vi "1_Waveform_Signal_Regression_Multi_Output(Training).vi"() -> ()   [LabVIEW 2020]
uses:
  <vilib>/Ngene/DeepLTK/Toolkit/NN_Train/Controls/NN_LR_Policy_Cfg.ctl
  <vilib>/Ngene/DeepLTK/Toolkit/NN_Train/Controls/NN_LR_Policy_Type.ctl
  <vilib>/Ngene/DeepLTK/Toolkit/NN_Train/Controls/NN_Train_Session_Data.ctl
  <vilib>/Ngene/DeepLTK/Toolkit/NN_Train/Controls/NN_Train_Params.ctl
  <vilib>/Ngene/DeepLTK/Toolkit/NN_Train/Controls/NN_Train_Optimizer.ctl
  <vilib>/Ngene/DeepLTK/Toolkit/NN_Train/Controls/NN_Train_Data_Sampling.ctl
  <vilib>/Ngene/DeepLTK/Toolkit/NN_Network/Controls/NN_Device.ctl
  <vilib>/Ngene/DeepLTK/Toolkit/NN_Layers/Layers/Input/Controls/NN_Layer_Config(Input1D).ctl
  <vilib>/Ngene/DeepLTK/Toolkit/NN_Layers/Layers/FC/Controls/NN_Layer_Config(FC).ctl
  <vilib>/Ngene/DeepLTK/Toolkit/NN_Activations/Controls/NN_Activation_Type.ctl
  <vilib>/Ngene/DeepLTK/Toolkit/NN_Layers/Controls/NN_Layer_Init_Params.ctl
  <vilib>/Ngene/DeepLTK/Toolkit/NN_Layers/Controls/NN_Layer_Weight_Init_Type.ctl
  <vilib>/Ngene/DeepLTK/Toolkit/NN_Network/Controls/NN_Save_Before_Destroy_Options.ctl
  <vilib>/Ngene/DeepLTK/Toolkit/NN_Layers/Layers/Input/NN_Layer_Create(Input1D).vi
  <vilib>/Ngene/DeepLTK/Toolkit/NN_Layers/Layers/FC/NN_Layer_Create(FC).vi
  <vilib>/Ngene/DeepLTK/Toolkit/NN_Train/Loss_Functions/NN_Set_Loss(MSE).vi
  <vilib>/Ngene/DeepLTK/Toolkit/NN_Network/subVIs/NN_Predict/NN_Predict(In1D_Out1D).vi
  <vilib>/Ngene/DeepLTK/Toolkit/NN_Train/Eval_Loss/NN_Eval_Test_Error_Loss/NN_Eval(In1D_Out1D).vi
  <vilib>/Ngene/DeepLTK/Toolkit/Deep_Learning_Toolkit_by_Ngene.lvlib
  <vilib>/ptbypt/NI_PtbyPt.lvlib
panel:
  out "Training Loss":sgl=0.0060925223 format="%#.6g"
  in  "Eval":bool
  out "Loss Graphs":cluster{"mean":dbl, "mean":dbl}(graph)={"mean"=0.014923217580653727, "mean"=0.03191827982664108}
  in  "NN_Device":T1=enum."GPU"
  out "Test Loss":sgl=0.03191828 format="%#.6g"
  in  "Stop Training":bool
  in  "NN_Train_Params":T2={"Optimizer"=enum."Adam", "Beta_1"=0.9, "Beta_2"=0.999, "Weight Decay(L1)"=1e-08, "Weight Decay(L2)"=1e-08, "Data_Sampling"=enum."Random"}
  out "Session Data":T5={"Epochs"=39.18592, "Tot_Iter"=30614, "LR"=6.25e-05, "LR_iter"=30615} {"LR" format="%#_3g"}
  in  "LR Update Policy":T6={"Policy_Type"=enum."Step", "LR0"=0.001, "k"=5.0, "WarmUp_Policy"=enum."Ramp", "WarmUp_Iter"=1000, "WarmUp_Ratio"=100.0} {"WarmUp_Ratio" min=1; "WarmUp_Iter" min=1; "LR0" format="%.7f"}
  # "Overview: This example demonstrates the usage of Deep Learning Toolkit for solving multiple output waveform signal regression problem. Specifically, a model is trained to predict multiple characteristic properties of a waveform, such as frequency, amplitude, phase, and DC offset..\nRequirements: DeepLTK - Deep Learning Toolkit for LabVIEW.\nInstructions:\n1.  Run the VI with current configuration of the training parameters and Learning Rate update policy.\n2. Observe how the training loss is decreasing.\n3. Press the \"Stop Training\" when the loss is not decreasing any more.\nMore Examples:  https://github.com/ngenehub/deepltk_examples"
  # "Waveform Signal Regression (Frequency Prediction) - Training"
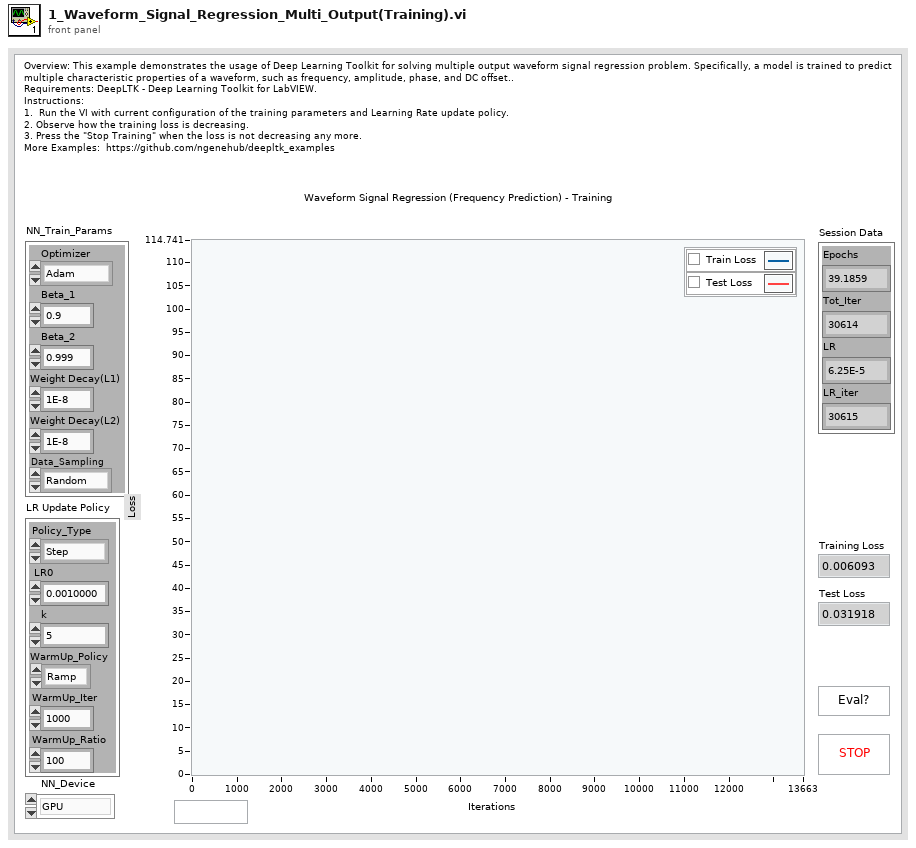
[diagram p1: front panel]
types:
  T1 = typedef "Deep_Learning_Toolkit_by_Ngene.lvlib/NN_Device.ctl" = enum16{"CPU", "GPU"}
  T2 = typedef "Deep_Learning_Toolkit_by_Ngene.lvlib/NN_Train_Params.ctl" = cluster{"Optimizer":T3, "Beta_1":sgl, "Beta_2":sgl, "Weight Decay(L1)":sgl, "Weight Decay(L2)":sgl, "Data_Sampling":T4}
  T3 = typedef "Deep_Learning_Toolkit_by_Ngene.lvlib/NN_Train_Optimizer.ctl" = enum16{"SGD", "Adam", "Adagrad", "Adadelta", "RMSProp", "Nesterov"}
  T4 = typedef "Deep_Learning_Toolkit_by_Ngene.lvlib/NN_Train_Data_Sampling.ctl" = enum16{"Random", "Sequential"}
  T5 = typedef "Deep_Learning_Toolkit_by_Ngene.lvlib/NN_Train_Session_Data.ctl" = cluster{"Epochs":sgl, "Tot_Iter":i32, "LR":sgl, "LR_iter":i32}
  T6 = typedef "Deep_Learning_Toolkit_by_Ngene.lvlib/NN_LR_Policy_Cfg.ctl" = cluster{"Policy_Type":T7, "LR0":dbl, "k":sgl, "WarmUp_Policy":enum16{"Step", "Ramp"}, "WarmUp_Iter":i32, "WarmUp_Ratio":sgl}
  T7 = typedef "Deep_Learning_Toolkit_by_Ngene.lvlib/NN_LR_Policy_Type.ctl" = enum16{"Manual", "Step", "Exp", "1/t"}
  T8 = typedef "Deep_Learning_Toolkit_by_Ngene.lvlib/NN_Layer_Config(FC).ctl" = cluster{"Name":string, "Size":i32, "BN":bool, "Activation":T9, "Init_Params":T10, "Custom_Params":string}
  T9 = typedef "Deep_Learning_Toolkit_by_Ngene.lvlib/NN_Activation_Type.ctl" = enum16{"Sigmoid", "ReLU", "LReLU", "ReLU6", "tanh", "Swish", "Mish", "None"}
  T10 = typedef "Deep_Learning_Toolkit_by_Ngene.lvlib/NN_Layer_Init_Params.ctl" = cluster{"Init_Type":T11, "Value":sgl}
  T11 = typedef "Deep_Learning_Toolkit_by_Ngene.lvlib/NN_Layer_Weight_Init_Type.ctl" = enum16{"Const", "Uniform", "Gaussian", "Xavier"}
  T12 = typedef "Deep_Learning_Toolkit_by_Ngene.lvlib/NN_Save_Before_Destroy_Options.ctl" = cluster{"CFG?":bool, "Weights?":bool, "Render?":bool}
  T13 = typedef "Deep_Learning_Toolkit_by_Ngene.lvlib/NN_Layer_Config(Input1D).ctl" = cluster{"Name":string, "Size":i32}
  T14 = typedef "Deep_Learning_Toolkit_by_Ngene.lvlib/NN_DataSets_All(In1D_Out1D).ctl" = cluster{"Train":T15, "Validation":T15, "Test":T15}
  T15 = typedef "Deep_Learning_Toolkit_by_Ngene.lvlib/NN_DataSet(In1D_Out1D).ctl" = cluster{"Inputs Ref.":T16, "Outputs Ref.":T16, "Dims_In":i32, "Dataset_Size":i32, "Outputs_idx Ref.":T17, "Dims_Out":i32, "Labels":string[], "File Paths":path[]}
  T16 = typedef "Deep_Learning_Toolkit_by_Ngene.lvlib/NN_Data_ref(2D_SGL).ctl" = refnum<data-value>
  T17 = typedef "Deep_Learning_Toolkit_by_Ngene.lvlib/NN_Data_ref(1D_I32).ctl" = refnum<data-value>
  T18 = typedef "Deep_Learning_Toolkit_by_Ngene.lvlib/NN.ctl" = cluster{"Name":string, "No of Layers":i32, "mBatch":i32, "Layers":T19[], "Dimty":T20, "Dims_In":T21, "Dims_Out":T21, "Working_Dir":path, "Train?":bool, "Train_Params":T2, "LR_Update_Policy":T6, "Session Data":T5, "Ground_truth":T22, "NNg_hdls":T23, "NN_Device":T1, "GPU Id":i32, "Labels":string[], "Receptive Field":T24[], "Loss_Type":T25, "Loss_Cfg_Prms":variant}
  T19 = typedef "Deep_Learning_Toolkit_by_Ngene.lvlib/NN_Layer_ref.ctl" = refnum<data-value>
  T20 = typedef "Deep_Learning_Toolkit_by_Ngene.lvlib/NN_In_Out_Dim-ty.ctl" = enum8{"In1D_Out1D", "In3D_Out1D", "In3D_Out3D", "In3D_OutBBox"}
  T21 = typedef "Deep_Learning_Toolkit_by_Ngene.lvlib/NN_Dims(C,H,W).ctl" = cluster{"C":i32, "H":i32, "W":i32}
  T22 = typedef "Deep_Learning_Toolkit_by_Ngene.lvlib/NN_Ground_truth.ctl" = cluster{"Y":variant, "Y_idx":T17}
  T23 = typedef "Deep_Learning_Toolkit_by_Ngene.lvlib/nng_cuda_handles.ctl" = cluster{"cudnn":u64, "cublas":u64, "stream":u64, "curand":u64}
  T24 = typedef "Deep_Learning_Toolkit_by_Ngene.lvlib/NN_Dims(V,H).ctl" = cluster{"V":i32, "H":i32}
  T25 = typedef "Deep_Learning_Toolkit_by_Ngene.lvlib/NN_Loss_Type.ctl" = enum16{"None", "MSE", "CrossEntropy", "YOLO_v2"}
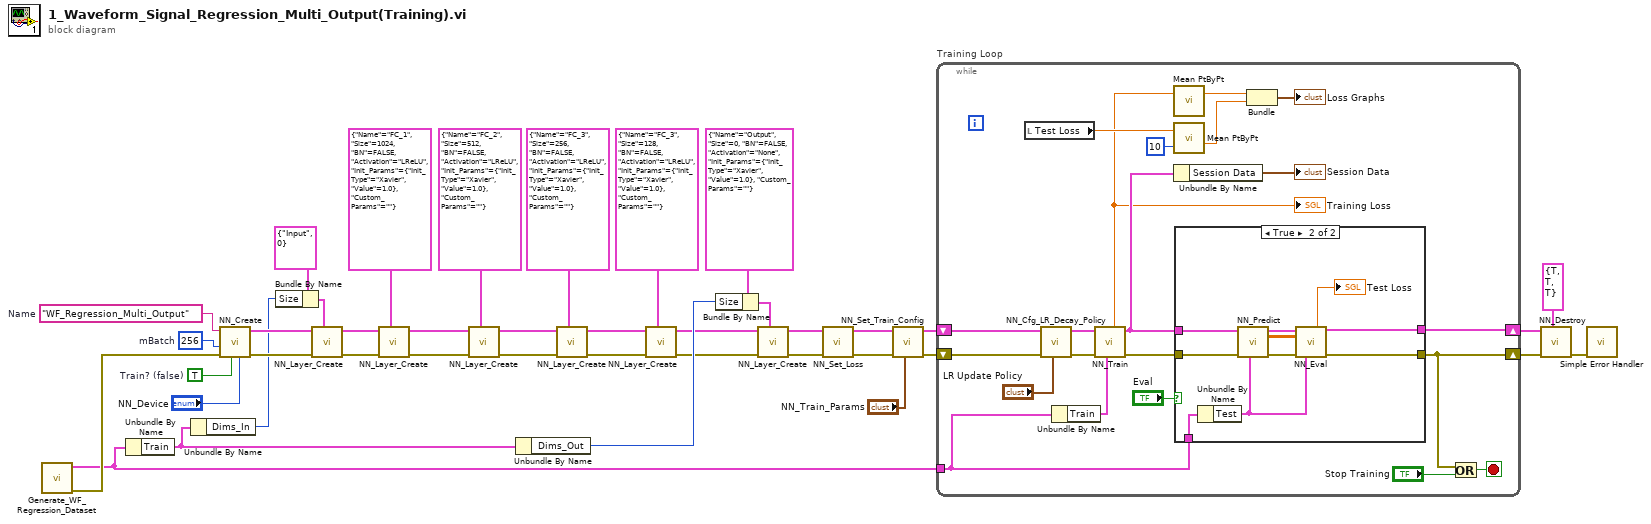
[diagram p0: block diagram]
diagram:
  w21 = "WF_Regression_Multi_Output"  # Name
  w22 = 256  # mBatch
  w23 = TRUE  # Train? (false)
  n1 = call "Generate_WF_Regression_Dataset.vi"() -> ("error out"=w32:errorcluster, "DataSets_All(In1D_Out1D)"=w8:T14)  [unwired: 10 in]
  n2 = Unbundle By Name(w8) -> ("Train"=w6:T15)
  n3 = Unbundle By Name(w6) -> ("Dims_In"=w30:i32)
  n4 = call <vilib>:"NN_Create.vi"("NN_Device"="NN_Device", "Train? (false)"=w23, "error in (no error)"=w32, "mBatch (1)"=w22, "Name"=w21) -> ("error out"=w39:errorcluster, "NN out"=w40:T18)  [unwired: 5 in]
  n5 = Bundle By Name(cluster=T13 {"Name"="Input", "Size"=0} ("Input1D_Cfg"), "Size"=w30) -> (w31:T13)
  n6 = call-poly <vilib>:"NN_Layer_Create.vi"("Input1D_Cfg"=w31, "error in (no error)"=w39, "NN in"=w40) -> ("error out"=w26:errorcluster, "NN out"=w27:T18)  [unwired: 6 in, 1 out]
  n7 = call-poly <vilib>:"NN_Layer_Create.vi"("FC_Cfg"=T8 {"Name"="FC_1", "Size"=1024, "BN"=FALSE, "Activation"=enum."LReLU", "Init_Params"={"Init_Type"=enum."Xavier", "Value"=1.0}, "Custom_Params"=""} ("FC_Cfg_1"), "error in (no error)"=w26, "NN in"=w27) -> ("error out"=w15:errorcluster, "NN out"=w16:T18)  [unwired: 6 in, 1 out]
  n8 = call-poly <vilib>:"NN_Layer_Create.vi"("FC_Cfg"=T8 {"Name"="FC_2", "Size"=512, "BN"=FALSE, "Activation"=enum."LReLU", "Init_Params"={"Init_Type"=enum."Xavier", "Value"=1.0}, "Custom_Params"=""} ("FC_Cfg_1"), "error in (no error)"=w15, "NN in"=w16) -> ("error out"=w11:errorcluster, "NN out"=w12:T18)  [unwired: 6 in, 1 out]
  n9 = Unbundle By Name(w6) -> ("Dims_Out"=w28:i32)
  n10 = call-poly <vilib>:"NN_Layer_Create.vi"("FC_Cfg"=T8 {"Name"="FC_3", "Size"=256, "BN"=FALSE, "Activation"=enum."LReLU", "Init_Params"={"Init_Type"=enum."Xavier", "Value"=1.0}, "Custom_Params"=""} ("FC_Cfg_1"), "error in (no error)"=w11, "NN in"=w12) -> ("error out"=w3:errorcluster, "NN out"=w4:T18)  [unwired: 6 in, 1 out]
  n11 = call-poly <vilib>:"NN_Layer_Create.vi"("FC_Cfg"=T8 {"Name"="FC_3", "Size"=128, "BN"=FALSE, "Activation"=enum."LReLU", "Init_Params"={"Init_Type"=enum."Xavier", "Value"=1.0}, "Custom_Params"=""} ("FC_Cfg_1"), "error in (no error)"=w3, "NN in"=w4) -> ("error out"=w1:errorcluster, "NN out"=w2:T18)  [unwired: 6 in, 1 out]
  n12 = Bundle By Name(cluster=T8 {"Name"="Output", "Size"=0, "BN"=FALSE, "Activation"=enum."None", "Init_Params"={"Init_Type"=enum."Xavier", "Value"=1.0}, "Custom_Params"=""} ("FC_Cfg_1"), "Size"=w28) -> (w29:T8)
  n13 = call-poly <vilib>:"NN_Layer_Create.vi"("FC_Cfg"=w29, "error in (no error)"=w1, "NN in"=w2) -> ("error out"=w35:errorcluster, "NN out"=w36:T18)  [unwired: 6 in, 1 out]
  n14 = call-poly <vilib>:"NN_Set_Loss.vi"("error in (no error)"=w35, "NN in"=w36) -> ("error out"=w18:errorcluster, "NN out"=w19:T18)  [unwired: 8 in]
  n15 = call <vilib>:"NN_Set_Train_Config.vi"("NN_Train_Params"="NN_Train_Params", "error in (no error)"=w18, "NN in"=w19) -> ("error out"=w24:errorcluster, "NN out"=w25:T18)  [unwired: 7 in]
  n16 = while "Training Loop" {
    shift-right: [w46] -> w9
    shift-left: w24 -> [w56]
    shift-right: [w52] -> w10
    shift-left: w25 -> [w59]
    tunnel: w8 -> [w42]
    stop <- w47 stop-if-true
    n17 = local read "Test Loss"() -> (w50:sgl)
    n18 = call <vilib>:"NN_Cfg_LR_Decay_Policy.vi"("LR_Decay_Params"="LR Update Policy", "error in (no error)"=w56, "NN in"=w59) -> ("error out"=w57:errorcluster, "NN out"=w58:T18)  [unwired: 7 in]
    n19 = Unbundle By Name(w42) -> ("Train"=w41:T15)
    n20 = call <vilib>:"NN_Train.vi"("Train Dataset"=w41, "error in (no error)"=w57, "NN in"=w58) -> ("error out"=w53:errorcluster, "NN out"=w54:T18, "Loss"=w48:sgl)  [unwired: 5 in, 1 out]
    "Training Loss" <- w48
    n21 = call <vilib>:"Mean PtByPt.vi"("x"=w48) -> ("mean"=w44:dbl)  [unwired: 3 in, 1 out]
    n22 = call <vilib>:"Mean PtByPt.vi"("x"=w50, "sample length"=10) -> ("mean"=w45:dbl)  [unwired: 2 in, 1 out]
    n23 = Unbundle By Name(w54) -> ("Session Data"=→"Session Data":T5)
    n24 = case shown="True" "Eval" {
      tunnel: w54 -> [w63 w72]
      tunnel: w53 -> [w62 w71]
      tunnel: [w63 w70] -> w52
      tunnel: [w62 w66] -> w46
      tunnel: w42 -> [_ w65]
      frame False {
      }
      frame True {
        n25 = Unbundle By Name(w65) -> ("Test"=w64:T15)
        n26 = call-poly <vilib>:"NN_Predict.vi"("Dataset"=w64, "error in (no error)"=w71, "NN in"=w72) -> ("error out"=w73:errorcluster, "Predictions"=w67:sgl[][], "NN out"=w68:T18)  [unwired: 6 in]
        n27 = call-poly <vilib>:"NN_Eval.vi"("NN in"=w68, "Predictions"=w67, "error in (no error)"=w73, "Dataset"=w64) -> ("Loss"=→"Test Loss":sgl, "NN out"=w70:T18, "error out"=w66:errorcluster)  [unwired: 7 in, 2 out]
      }
    }
    n28 = Bundle("mean"=w44, "mean"=w45) -> (→"Loss Graphs":cluster{"mean":dbl, "mean":dbl})  [unwired: 1 in]
    n29 = Or(x=w46, y="Stop Training") -> (x .or. y?=w47:bool)
  }
  n30 = call <vilib>:"NN_Destroy.vi"("Save (T, T, T)"=T12 {"CFG?"=TRUE, "Weights?"=TRUE, "Render?"=TRUE}, "error in (no error)"=w9, "NN in"=w10) -> ("error out"=w34:errorcluster)  [unwired: 8 in]
  n31 = call <vilib>:"Simple Error Handler.vi"("error in (no error)"=w34) -> ()  [unwired: 4 in, 5 out]
